vi "Bridge Read.vi"(8 "error in (no error)":errorcluster, 10 "multiline":u16(ring) items=["Single Line", "Multi-Line"], 11 "VISA resource name":refnum<visa-resource-name>) -> (0 "error out":errorcluster, 2 "read buffer":string, 3 "VISA resource name out":refnum<visa-resource-name>)   [LabVIEW 2024, in "Andeen-Hagerling 2700A.lvlib"]
doc: "Wrapper VI for the VISA read. Will read multiline serial results if multiline parameter is set. Adjusts formatting to make GPIB and serial results identical."
uses:
  Andeen-Hagerling 2700A.lvlib
  <vilib>/Utility/error.llb/Trim Whitespace One-Sided.vi
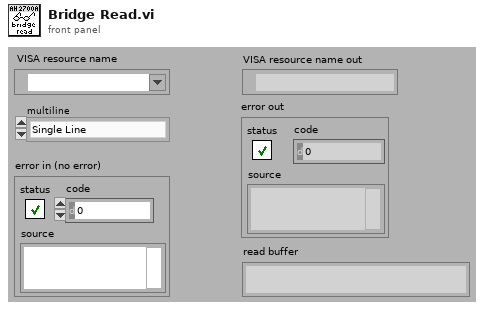
[diagram p1: front panel]
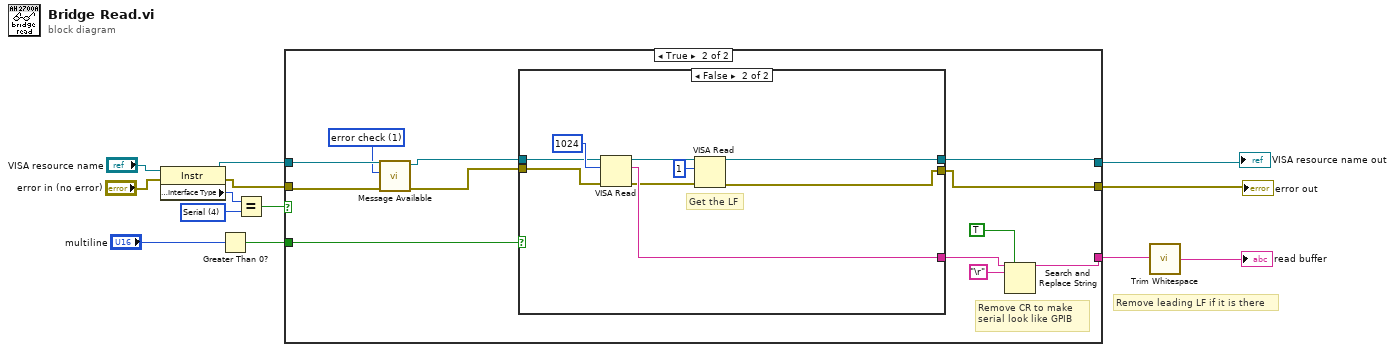
[diagram p0: block diagram]
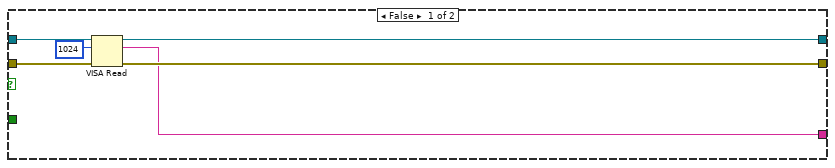
[diagram p2: hidden frame]
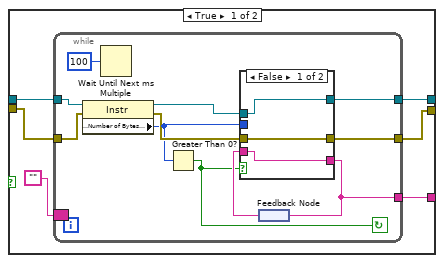
[diagram p3: hidden frame]
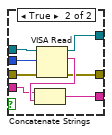
[diagram p4: hidden frame]
diagram:
  w13 = u16 4 items=["GPIB"=1, "VXI"=2, "GPIB-VXI"=3, "Serial"=4, "PXI"=5, "TCPIP"=6, "USB"=7] ("Interface Information:Interface Type")
  # "Remove leading LF if it is there"
  n1 = property class="Instr"(reference="VISA resource name", error in="error in (no error)") -> (reference out=w8:refnum<visa-resource-name>, error out=w7:errorcluster, "Interface Information:Interface Type"=w12:u16)
  n2 = Greater Than 0?(x="multiline") -> (x > 0?=w3:bool)
  n3 = Equal?(x=w12, y=w13) -> (x = y?=w9:bool)
  n4 = case shown="True" w9 {
    tunnel: w8 -> [w18 w25]
    tunnel: w7 -> [w17 w22]
    tunnel: [w16 w30] -> w6
    tunnel: [w15 w29] -> w5
    tunnel: [w14 w26] -> w2
    tunnel: w3 -> [_ w31]
    frame False {
      n5 = VISA Read(VISA resource name=w18, byte count=u32 1024, error in (no error)=w17) -> (VISA resource name out=w16:refnum<visa-resource-name>, read buffer=w14:string, error out=w15:errorcluster)  [unwired: 1 out]
    }
    frame True {
      w21 = u16 1 items=["none", "error check", "multiline read", "infinite"] ("delay")
      # "Remove CR to make \nserial look like GPIB"
      n6 = call "Message Available.vi"("error in (no error)"=w22, "delay"=w21, "VISA resource name"=w25) -> ("error out"=w23:errorcluster, "VISA resource name out"=w24:refnum<visa-resource-name>)  [unwired: 6 in, 1 out]
      n7 = case shown="False" w31 {
        tunnel: w24 -> [w37 w66]
        tunnel: w23 -> [w36 w65]
        tunnel: [w35 w60] -> w30
        tunnel: [w34 w62] -> w29
        tunnel: [w32 w67] -> w28
        frame True {
          n8 = while {
            tunnel: w37 -> [w46]
            tunnel: w36 -> [w45]
            tunnel: [w42] -> w35
            tunnel: [w41] -> w34
            tunnel: [w47] -> w32
            border: "" -> [_]
            stop <- w38 continue-if-true
            n9 = property class="Instr"(reference=w46, error in=w45) -> (reference out=w44:refnum<visa-resource-name>, error out=w43:errorcluster, "Serial Settings:Number of Bytes at Serial Port"=w39:u32)
            n10 = Wait Until Next ms Multiple(millisecond multiple=u32 100) -> ()  [unwired: 1 out]
            n11 = Greater Than 0?(x=w39) -> (x > 0?=w38:bool)
            n12 = feedback #1() -> (w48:string)
            n13 = case shown="False" w38 {
              tunnel: w48 -> [w51 w58]
              tunnel: [w51 w57] -> w47
              tunnel: w44 -> [w49 w56]
              tunnel: w43 -> [w50 w55]
              tunnel: [w49 w54] -> w42
              tunnel: [w50 w53] -> w41
              tunnel: w39 -> [_ w52]
              frame False {
              }
              frame True {
                n14 = VISA Read(VISA resource name=w56, byte count=w52, error in (no error)=w55) -> (VISA resource name out=w54:refnum<visa-resource-name>, read buffer=w59:string, error out=w53:errorcluster)  [unwired: 1 out]
                n15 = Concatenate Strings(w58, w59) -> (w57:string)
              }
            }
            n16 = feedback-in #1(w47) -> ()
          }
        }
        frame False {
          # "Get the LF"
          n17 = VISA Read(VISA resource name=w66, byte count=u32 1024, error in (no error)=w65) -> (VISA resource name out=w64:refnum<visa-resource-name>, read buffer=w67:string, error out=w63:errorcluster)  [unwired: 1 out]
          n18 = VISA Read(VISA resource name=w64, byte count=u32 1, error in (no error)=w63) -> (VISA resource name out=w60:refnum<visa-resource-name>, error out=w62:errorcluster)  [unwired: 2 out]
        }
      }
      n19 = Search and Replace String(replace all?=TRUE ("replace all? (F)"), input string=w28, search string="\r") -> (result string=w26:string)  [unwired: 5 in, 3 out]
    }
  }
  "error out" <- w5
  "VISA resource name out" <- w6
  n20 = call <vilib>:"Trim Whitespace.vi"("string"=w2) -> ("trimmed string"=→"read buffer":string)  [unwired: 1 in]
